vi "Actor Core.vi"(8 "error in":errorcluster, 11 "SensorViewSmall in":refnum<class "SensorViewSmall.lvclass">) -> (0 "error out":errorcluster, 3 "Actor out":refnum<class "Actor.lvclass">)   [LabVIEW 2012, in "Sensor Definition.lvlib" / "SensorViewSmall.lvclass"]
doc: "(<B>Filename</B>: Actor Framework.lvlib:Actor.lvclass:Actor Core.vi)\n\nReceives messages to the actor, reacts to them, and initiates any error handling that may shut the actor down.\n\nDescendant classes may override this VI to append parallel tasks for the actor to complete while it handles messages. Overrides use the Call Parent Method node."
uses:
  SensorViewSmall.lvclass
  <vilib>/ActorFramework/Actor/Actor.lvclass
  Controls/String XControl/String XControl.xctl
  SensorView.lvclass
  <vilib>/ActorFramework/Actor/Actor.lvclass/Actor.ctl
  Win8uiFramework/ViewableActor.lvclass/ViewableActor.ctl
  SensorView.lvclass/SensorView.ctl
  SensorInfo.lvclass/SensorInfo.ctl
  SensorData.lvclass
  <vilib>/ActorFramework/Message Enqueuer/Message Enqueuer.lvclass/Message Enqueuer.ctl
  SensorInfo/Read Name.vi
  SensorInfo/Read Description.vi
  Win8uiFramework/Read Stop Event.vi
  SensorView/Read SensorInfo Changed Event.vi
  SensorView/Read SensorData Changed Event.vi
  SensorView/Read SensorInfo.vi
  <vilib>/ActorFramework/Message Enqueuer/Enqueue.vi
  <vilib>/ActorFramework/Message Priority Queue/Priority Enqueue.vi
  SensorInfo.lvclass
  Sensor Messages/Launch Detail View Msg/Launch Detail View Msg.lvclass
  Win8uiFramework/ViewableActor.lvclass
  Win8uiFramework/Win8uiFramework.lvlib
panel:
  out "Thumbnail Chart":dbl(graph)
  out "String XControl":string(xcontrol)
  out "Tank":dbl(slide) scale=0.0..1.0 scale format="%_2f"
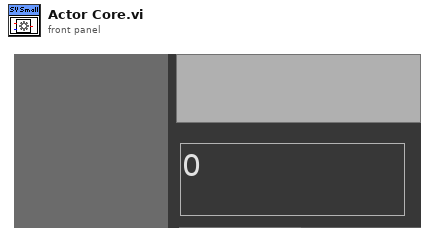
[diagram p1: front panel]
types:
  T1 = cluster{"horizontal":enum16{"left", "center", "right"}, "vertical":enum16{"top", "center", "bottom"}}
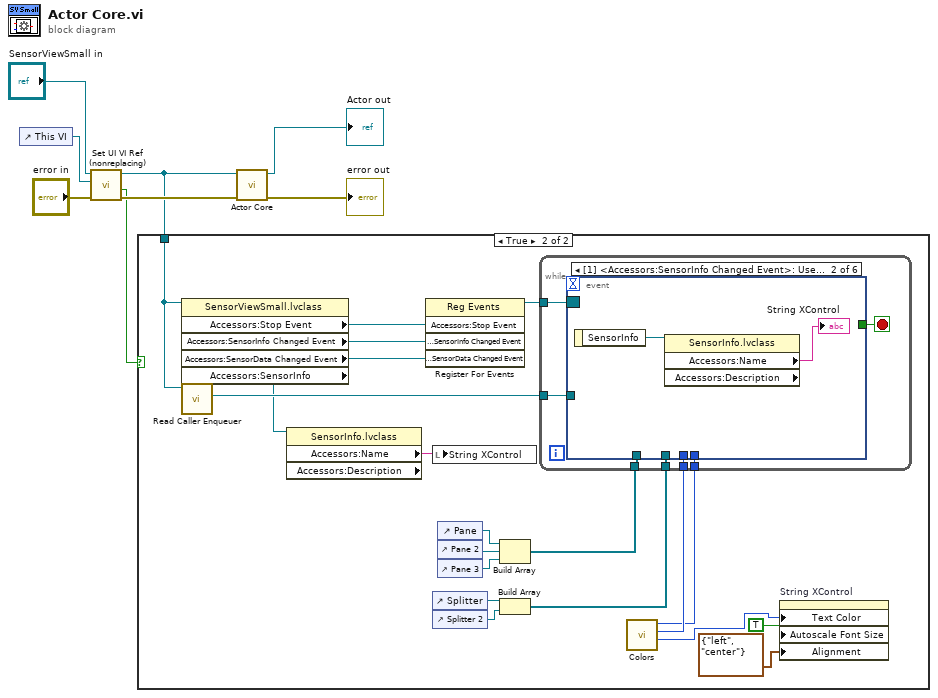
[diagram p0: block diagram]
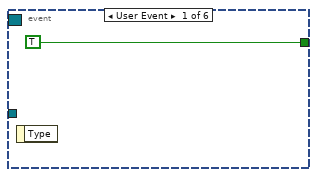
[diagram p3: hidden frame]
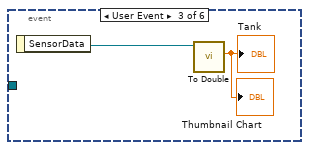
[diagram p4: hidden frame]
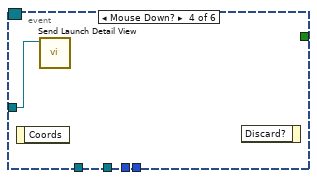
[diagram p5: hidden frame]
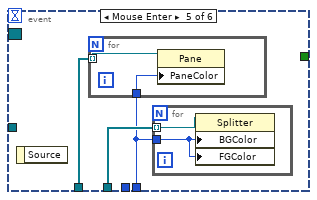
[diagram p6: hidden frame]
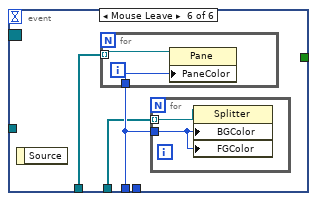
[diagram p7: hidden frame]
diagram:
  n1 = control-ref of="This VI"() -> (w3:refnum<vi>)
  n2 = call "Set UI VI Ref (nonreplacing).vi"("error in (no error)"="error in", "UI VI Ref"=w3, "ViewableActor in"="SensorViewSmall in") -> ("error out"=w4:errorcluster, "Top Level UI?"=w2:bool, "ViewableActor out"=w1:refnum<class "SensorViewSmall.lvclass">)  [unwired: 6 in]
  n3 = case shown="True" w2 {
    tunnel: w1 -> [_ w24]
    frame False {
    }
    frame True {
      n4 = property class="SensorViewSmall.lvclass"(reference=w24) -> ("Accessors:Stop Event"=w28:refnum<user-event>, "Accessors:SensorInfo Changed Event"=w27:refnum<user-event>, "Accessors:SensorData Changed Event"=w25:refnum<user-event>, "Accessors:SensorInfo"=w13:refnum<class "SensorInfo.lvclass">)  [unwired: 1 in, 2 out]
      n5 = call <vilib>:"Read Caller Enqueuer.vi"("Actor"=w24) -> ("Caller Enqueuer"=w23:refnum<class "Message Enqueuer.lvclass">)  [unwired: 10 in]
      n6 = property class="SensorInfo.lvclass" props=["Accessors:Name", "Accessors:Description"](reference=w13) -> ("Accessors:Name"=w12:string)  [unwired: 1 in, 3 out]
      n7 = register-events(w28, w27, w25) -> (reference out=w26:refnum<event-registration>)  [unwired: 2 in, 1 out]
      n8 = local write "String XControl"(w12) -> ()
      n9 = control-ref of="Splitter"() -> (w18:refnum<vi>)
      n10 = control-ref of="Splitter 2"() -> (w17:refnum<vi>)
      n11 = control-ref of="Pane"() -> (w20:refnum<vi>)
      n12 = control-ref of="Pane 2"() -> (w21:refnum<vi>)
      n13 = control-ref of="Pane 3"() -> (w22:refnum<vi>)
      n14 = Build Array(w20, w21, w22) -> (w19:refnum<vi>[])
      n15 = Build Array(w18, w17) -> (w16:refnum<vi>[])
      n16 = call "Colors.vi"() -> ("Text Color"=w9:u32, "GridView Normal Color"=w11:u32, "GridView Mouseover Color"=w10:u32)  [unwired: 8 in, 1 out]
      n17 = while {
        tunnel: w26 -> [w35]
        tunnel: w23 -> [w33]
        tunnel: w19 -> [w32]
        tunnel: w10 -> [w31]
        tunnel: w11 -> [w30]
        tunnel: w16 -> [w29]
        stop <- w34 stop-if-true
        n18 = event shown="[1] <Accessors:SensorInfo Changed Event>: User Event" {
          selector: w35 -> [_ _ _ _ _ _]
          dyn-events: _ -> [_ _ _ _ _ _]
          timeout: _ -> [_ _ _ _ _ _]
          tunnel: [TRUE _ _ _ _ _] -> w34
          tunnel: w33 -> [_ _ _ w41 _ _]
          tunnel: w32 -> [_ _ _ _ w44 w51]
          tunnel: w31 -> [_ _ _ _ w42 _]
          tunnel: w30 -> [_ _ _ _ _ w50]
          tunnel: w29 -> [_ _ _ _ w43 w49]
          event User Event {
            n19 = event-data() -> ()  [unwired: 1 in, 1 out]
          }
          event User Event {
            n20 = event-data() -> ("SensorInfo"=w38:refnum<class "SensorInfo.lvclass">)  [unwired: 1 in]
            n21 = property class="SensorInfo.lvclass" props=["Accessors:Name", "Accessors:Description"](reference=w38) -> ("Accessors:Name"=→"String XControl":string)  [unwired: 1 in, 3 out]
          }
          event User Event {
            n22 = event-data() -> ("SensorData"=w39:refnum<class "SensorData.lvclass">)  [unwired: 1 in]
            n23 = call-dynamic "To Double.vi"("SensorData in"=w39) -> ("Value"=→"Tank" →"Thumbnail Chart":dbl)  [unwired: 8 in, 2 out]
          }
          event Mouse Down? {
            n24 = event-data() -> ()  [unwired: 1 in, 1 out]
            n25 = call "Send Launch Detail View.vi"("Message Enqueuer"=w41) -> ()  [unwired: 9 in, 2 out]
            n26 = event-data() -> ()  [unwired: 2 in, 1 out]
          }
          event Mouse Enter {
            n27 = event-data() -> ()  [unwired: 1 in, 1 out]
            n28 = for {
              tunnel: w44 -> [w48] mode=indexing
              tunnel: w42 -> [w47]
              n29 = property class="Pane"(reference=w48, "PaneColor"=w47) -> ()  [unwired: 1 in, 2 out]
            }
            n30 = for {
              tunnel: w43 -> [w46] mode=indexing
              tunnel: w42 -> [w45]
              n31 = property class="Splitter"(reference=w46, "BGColor"=w45, "FGColor"=w45) -> ()  [unwired: 1 in, 2 out]
            }
          }
          event Mouse Leave {
            n32 = event-data() -> ()  [unwired: 1 in, 1 out]
            n33 = for {
              tunnel: w51 -> [w55] mode=indexing
              tunnel: w50 -> [w54]
              n34 = property class="Pane"(reference=w55, "PaneColor"=w54) -> ()  [unwired: 1 in, 2 out]
            }
            n35 = for {
              tunnel: w49 -> [w53] mode=indexing
              tunnel: w50 -> [w52]
              n36 = property class="Splitter"(reference=w53, "BGColor"=w52, "FGColor"=w52) -> ()  [unwired: 1 in, 2 out]
            }
          }
        }
      }
      n37 = property on="String XControl" class="String XControl (strict)"("Text Color"=w9, "Autoscale Font Size"=TRUE, "Alignment"=T1 {"horizontal"=enum."left", "vertical"=enum."center"}) -> ()  [unwired: 2 in, 2 out]
    }
  }
  n38 = call-parent "Actor Core.vi"("error in"=w4, "Actor in"=w1) -> ("error out"=→"error out":errorcluster, "Actor out"=→"Actor out":refnum<class "Actor.lvclass">)  [unwired: 8 in]
